vi "Queue Send Message With Name.vi"(8 "error in (no error)":errorcluster caption="Error In", 9 "Data":variant, 10 "Message":string, 11 "VI Name":refnum<vi>) -> (0 "error out":errorcluster caption="Error Out", 3 "Queue Out":refnum<queue>)   [LabVIEW 2020]
uses:
  Queue Message.ctl
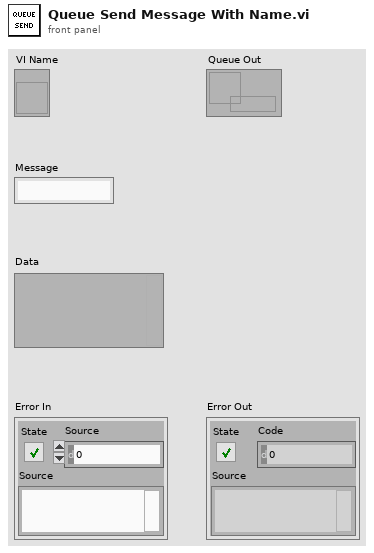
[diagram p1: front panel]
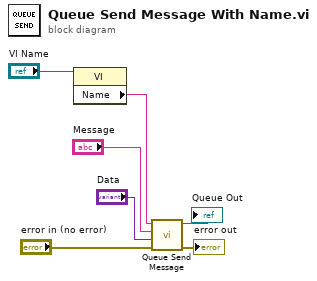
[diagram p0: block diagram]
diagram:
  n1 = property class="VI"(reference="VI Name") -> ("Name"=w6:string)  [unwired: 1 in, 2 out]
  n2 = call "Queue Send Message.vi"("error in (no error)"="error in (no error)", "Data"="Data", "Message"="Message", "Queue Name"=w6) -> ("error out"=→"error out":errorcluster, "Queue Out"=→"Queue Out":refnum<queue>)  [unwired: 5 in, 1 out]
